vi "Hot and Cold Gallons.vi"(11 "Data":string) -> (2 "ColdGallons":dbl, 3 "Hot Gallons":dbl)   [LabVIEW 2016, in "GEA2_Toolkit.lvlib"]
uses:
  library/GEA2_Toolkit.lvlib
panel:
  # "04 B3 04 9B"
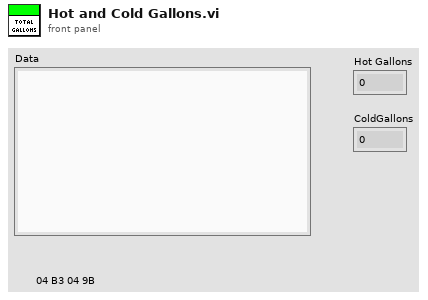
[diagram p1: front panel]
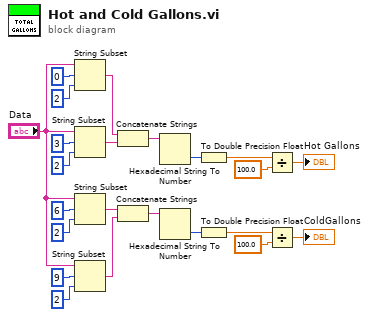
[diagram p0: block diagram]
diagram:
  n1 = String Subset(string="Data", offset (0)=0, length (rest)=2 ("length (rest)")) -> (substring=w5:string)
  n2 = String Subset(string="Data", offset (0)=3, length (rest)=2 ("length (rest)")) -> (substring=w6:string)
  n3 = String Subset(string="Data", offset (0)=6, length (rest)=2 ("length (rest)")) -> (substring=w17:string)
  n4 = String Subset(string="Data", offset (0)=9, length (rest)=2 ("length (rest)")) -> (substring=w16:string)
  n5 = Concatenate Strings(w5, w6) -> (w7:string)
  n6 = Concatenate Strings(w17, w16) -> (w15:string)
  n7 = Hexadecimal String To Number(string=w7) -> (number=w10:u32)  [unwired: 2 in, 1 out]
  n8 = Hexadecimal String To Number(string=w15) -> (number=w12:u32)  [unwired: 2 in, 1 out]
  n9 = To Double Precision Float(number=w10) -> (double precision float=w9:dbl)
  n10 = To Double Precision Float(number=w12) -> (double precision float=w13:dbl)
  n11 = Divide(x=w9, y=100.0) -> (x/y=→"Hot Gallons":dbl)
  n12 = Divide(x=w13, y=100.0) -> (x/y=→"ColdGallons":dbl)
